vi "PTSequencer.check step conditions.vi"(0 "i ref in":refnum<vi>, 3 "ms timeout (10000)":i32=10000, 5 "error in (no error)":errorcluster) -> (14 "i ref out":refnum<vi>, 16 "next state":string, 17 "timed out":bool, 19 "error out":errorcluster)   [LabVIEW 2014, in "PTSequencer.lvlib"]
uses:
  PTSequencer.lvlib
  CS_Core/BaseSM/BaseSM.lvlib
  CSlibraries-extern/DimLVEvent/LVDimInterface/LVDimInterface.lvlib
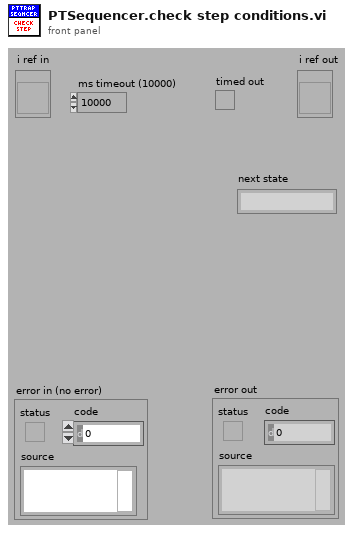
[diagram p1: front panel]
types:
  T1 = typedef "PTSequencer.lvlib/PTSequencer.i attribute.ctl" = cluster{"subsequence":bool, "mode":T2, "i step":i32, "nofLoops":i32, "i loop":i32, "Running":bool, "Paused":bool, "step done":bool, "loop done":bool, "seq done":bool, "DIM IDs":cluster{"step done":i32, "loop done":i32, "seq done":i32, "i step":i32, "i loop":i32}, "use stop conditions":bool, "stop conditions":T3[], "Step List":T5[], "DIM subsriptions":string[], "stop cond indexes":i32[], "step cond indexes":cluster{"step condition IDs":cluster{"step ID":i32, "condition ID":i32}[]}[], "Delay Start Time":timestamp, "status":string, "stopping":bool}
  T2 = typedef "PTSequencer.lvlib/PTSequencer.mode.ctl" = enum16{"single", "loop", "for loop"}
  T3 = typedef "PTSequencer.lvlib/PTSequencer.DIM service condition.ctl" = cluster{"DIM service":string, "descr":string, "nomValue":T4, "actValue":T4, "matched":bool, "DIM Status":cluster{"no link":bool, "quality":i32, "Time Stamp":timestamp}}
  T4 = typedef "CoreDefs.rawDataType.ctl" = i8[]
  T5 = typedef "PTSequencer.lvlib/PTSequencer.step.ctl" = cluster{"description":string, "object parameters":cluster{"object":string, "selector":string, "descriptor":string, "data":T4, "subsequence":bool, "call mode":enum16{"Simple DIM", "Synchronous"}, "data in":T4}, "result action":cluster{"check":bool, "passed":enum16{"Next", "Previous", "Repeat", "Jump"}, "failed":enum16{"Next", "Previous", "Repeat", "Jump"}, "jumpID_passed":i32, "jumpID_failed":i32}, "conditions":T3[], "fulfilled ":bool, "use delay":bool, "delay time (s)":dbl, "ID":i32}
  T6 = typedef "BaseSM.lvlib/BaseSM.i attribute.ctl" = cluster{"stateError":i32, "stateStatus":string, "stateQuality":T7, "ProcStateRef":refnum<vi>, "thread ref":refnum<vi>, "actState":string, "reqState":string, "SMQueue":refnum<queue>, "stateErrorID":i32, "stateStatusID":i32}
  T7 = typedef "BaseSM.lvlib/BaseSM.stateQuality.ctl" = i16
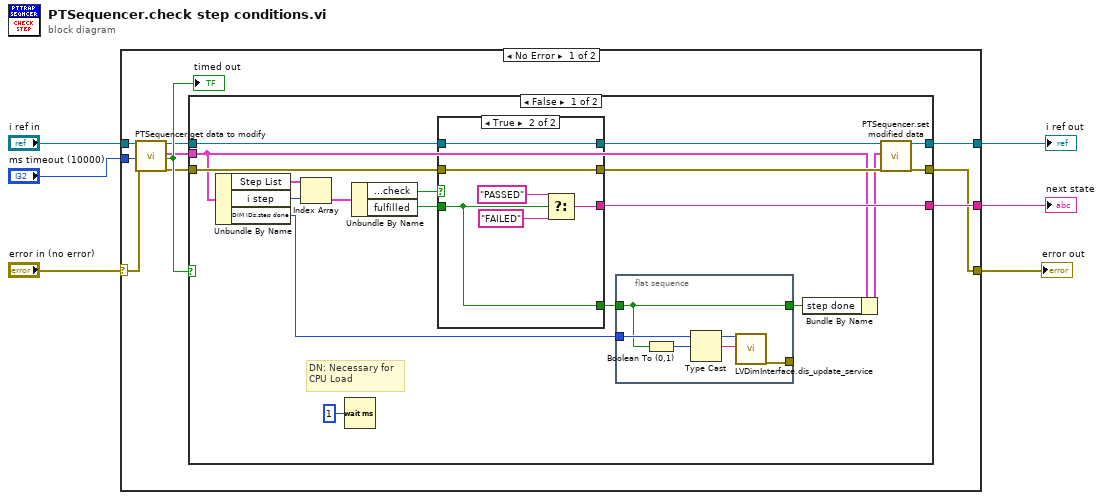
[diagram p0: block diagram]
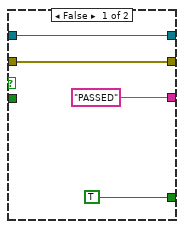
[diagram p2: hidden frame]
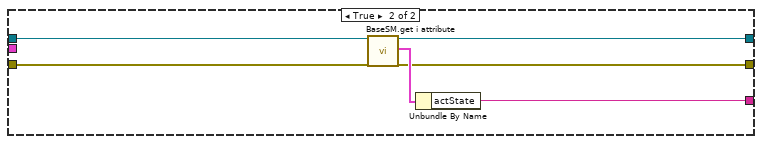
[diagram p3: hidden frame]
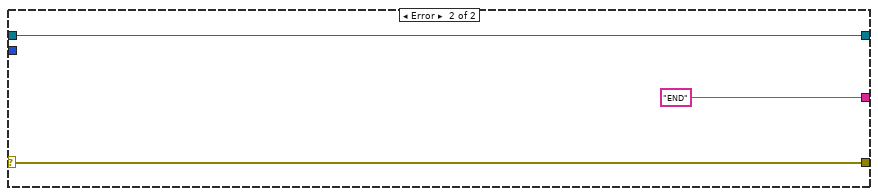
[diagram p4: hidden frame]
diagram:
  n1 = case shown="No Error" "error in (no error)" {
    selector: "error in (no error)" -> [w15 w58]
    tunnel: "i ref in" -> [w16 w57]
    tunnel: "ms timeout (10000)" -> [w13 _]
    tunnel: [w10 w57] -> w3
    tunnel: [w7 w58] -> w2
    tunnel: [w8 "END"] -> w1
    frame No Error {
      n2 = call "PTSequencer.get data to modify.vi"("i ref in"=w16, "ms timeout (10000)"=w13, "error in (no error)"=w15) -> ("i ref out"=w12:refnum<vi>, "i attribute"=w9:T1, "timed out"=w14:bool, "error out"=w11:errorcluster)  [unwired: 13 in]
      "timed out" <- w14
      n3 = case shown="False" w14 {
        tunnel: [w30 w52] -> w8
        tunnel: w12 -> [w29 w54]
        tunnel: w11 -> [w28 w53]
        tunnel: [w26 w51] -> w10
        tunnel: [w24 w50] -> w7
        tunnel: w9 -> [w18 _]
        frame False {
          # "DN: Necessary for\nCPU Load"
          n4 = Unbundle By Name(w18) -> ("Step List"=w34:T5[], "i step"=w33:i32, "DIM IDs.step done"=w22:i32)
          n5 = Index Array(array=w34, index=w33) -> (element=w32:T5)
          n6 = Wait (ms)(milliseconds to wait=u32 1) -> ()  [unwired: 1 out]
          n7 = Unbundle By Name(w32) -> ("result action.check"=w31:bool, "fulfilled"=w19:bool)
          n8 = case shown="True" w31 {
            tunnel: ["PASSED" w44] -> w30
            tunnel: w29 -> [w42 w46]
            tunnel: [w42 w46] -> w27
            tunnel: w28 -> [w41 w45]
            tunnel: [w41 w45] -> w25
            tunnel: [TRUE w47] -> w21
            tunnel: w19 -> [_ w47]
            frame False {
            }
            frame True {
              n9 = Select(t="PASSED", s=w47, f="FAILED") -> (s? t:f=w44:string)
            }
          }
          n10 = flat-sequence {
            tunnel: w22 -> [w37]
            tunnel: w21 -> [w36]
            tunnel: [w36] -> w20
            tunnel: [w35] -> _
            frame #0 {
              n11 = Boolean To (0,1)(Boolean=w36) -> (0, 1=w39:i16)
              n12 = Type Cast(x=w39) -> (*(type *) &x=w38:string)  [unwired: 1 in]
              n13 = call "LVDimInterface.dis_update_service.vi"("my_serviceID"=w37, "data"=w38) -> ("error out"=w35:errorcluster)  [unwired: 15 in, 2 out]
            }
          }
          n14 = Bundle By Name(cluster=w18, "step done"=w20) -> (w23:T1)
          n15 = call "PTSequencer.set modified data.vi"("i ref in"=w27, "CLASS.i attribute"=w23, "error in (no error)"=w25) -> ("i ref out"=w26:refnum<vi>, "error out"=w24:errorcluster)  [unwired: 15 in]
        }
        frame True {
          n16 = call "BaseSM.get i attribute.vi"("i ref in"=w54, "error in (no error)"=w53) -> ("i ref out"=w51:refnum<vi>, "i attribute"=w55:T6, "error out"=w50:errorcluster)  [unwired: 15 in]
          n17 = Unbundle By Name(w55) -> ("actState"=w52:string)
        }
      }
    }
    frame Error {
    }
  }
  "i ref out" <- w3
  "error out" <- w2
  "next state" <- w1
